vi "Globals.vi"() -> ()   [LabVIEW 2024]
uses:
  <vilib>/MediaMongrels Ltd/WebSockets/WebSockets/WebSocket Server/WebSocket Server.lvclass
panel:
  in  "WebSocket":refnum<class "WebSocket Server.lvclass">
  out "Network Stream Clock":u32
  out "Aborts Iteration Clock":u32
  out "Sequencing Iteration Clock":u32
  out "Controls Iteration Clock":u32
  out "Processing_Logging Iteration Clock":u32
  out "Acquisition Iteration Clock":u32
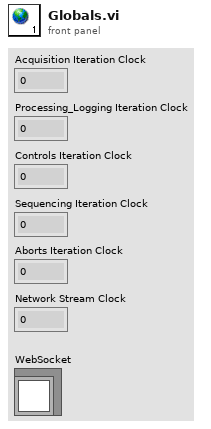
[diagram p1: front panel]
diagram:
